vi "FestoCPX.Valves(array).vi"(6 "Delay [ms] (50)":u32=50, 8 "error in (no error)":errorcluster, 9 "State":bool[](array[boolean]), 10 "Outputs":T1[](array[typedef])) -> (0 "error out":errorcluster)   [LabVIEW 2014]
uses:
  FestoCPX.DO.Signal.ctl
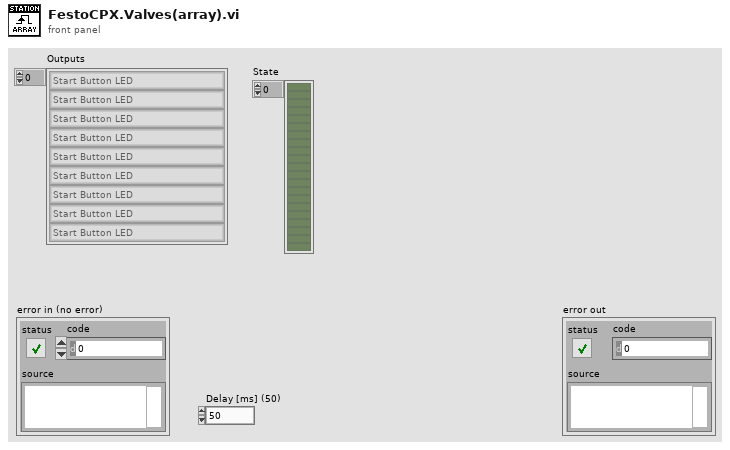
[diagram p1: front panel]
types:
  T1 = typedef "FestoCPX.DO.Signal.ctl" = enum16{"Start Button LED", "White Button LED", "Blue Button LED", "Red Button LED", "Safety Circuit Reset", "Air Main Valve", "Laser Interlock", "Traffic Light Red", "Traffic Light Orange", "Traffic Light Green", "Horn", "Q1 Vent B Work", "Q1 Vent B Home", "Q2 Vent A Work", "Q2 Vent A Home", "Q3 Product Press A Work", "Q3 Product Press A Home", "Q4 Product Press B Work", "Q4 Product Press B Home", "Q5 Pneumatic Connection A Work", "Q5 Pneumatic Connection A Home", "Q6 Pneumatic Connection B Work", "Q6 Pneumatic Connection B Home", "Q7 Laser Press Work", "Q7 Laser Press Home", "Q8 Table Lock Work", "Q8 Table Lock Home", "Q13 Table Turn Work", "Q13 Table Turn Home"}
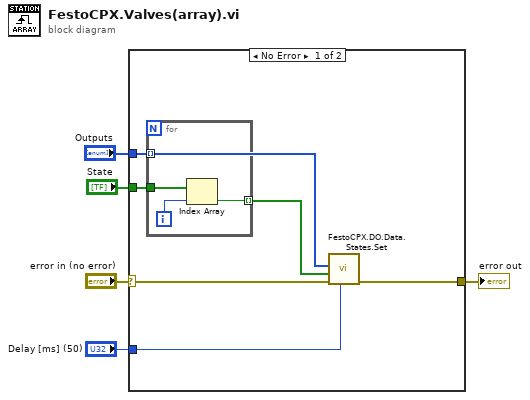
[diagram p0: block diagram]
diagram:
  n1 = case shown="No Error" "error in (no error)" {
    selector: "error in (no error)" -> [w11 w15]
    tunnel: [w10 w15] -> w5
    tunnel: "Delay [ms] (50)" -> [w6 _]
    tunnel: "Outputs" -> [w9 _]
    tunnel: "State" -> [w8 _]
    frame No Error {
      n2 = for {
        tunnel: w9 -> [_] mode=indexing
        tunnel: w8 -> [w14]
        tunnel: [w12] -> w7 mode=indexing
        i -> [w13]
        n3 = Index Array(array=w14, index=w13) -> (element=w12:bool)
      }
      n4 = call "FestoCPX.DO.Data.States.Set.vi"("Delay [ms] (0)"=w6, "error in (no error)"=w11, "State"=w7, "CPX.DO"=w9) -> ("error out"=w10:errorcluster)  [unwired: 7 in]
    }
    frame Error {
    }
  }
  "error out" <- w5
